vi "Config.vi"(8 "error in (no error)":errorcluster, 11 "SimSyA in":refnum<class "SimSyA.lvclass">) -> (0 "error out":errorcluster, 2 "HAL Config Data":T1, 3 "SimSyA out":refnum<class "SimSyA.lvclass">)   [LabVIEW 2014, in "SimSyA.lvlib" / "SimSyA.lvclass"]
uses:
  SimSyA.lvclass
  DriverMasterSync/build/DriverMasterSync.lvlibp/Modules/HAL/TypeDefs/HAL Config Data.ctl
  SimSyA.lvclass/SimSyA.ctl
  DriverMasterSync/build/DriverMasterSync.lvlibp/Modules/HAL/DriverMasterSync/DriverMasterSyncClass/DriverMasterSync.lvclass
  DriverMasterSync/build/DriverMasterSync.lvlibp
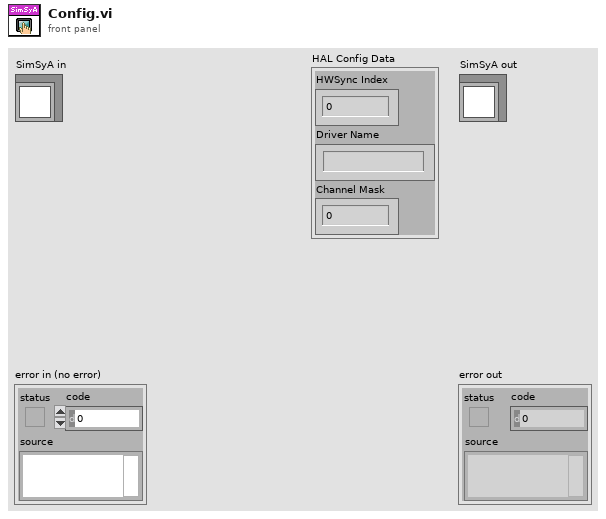
[diagram p1: front panel]
types:
  T1 = typedef "DriverMasterSync.lvlibp/HAL Config Data.ctl" = cluster{"HWSync Index":u32, "Driver Name":string, "Channel Mask":u64}
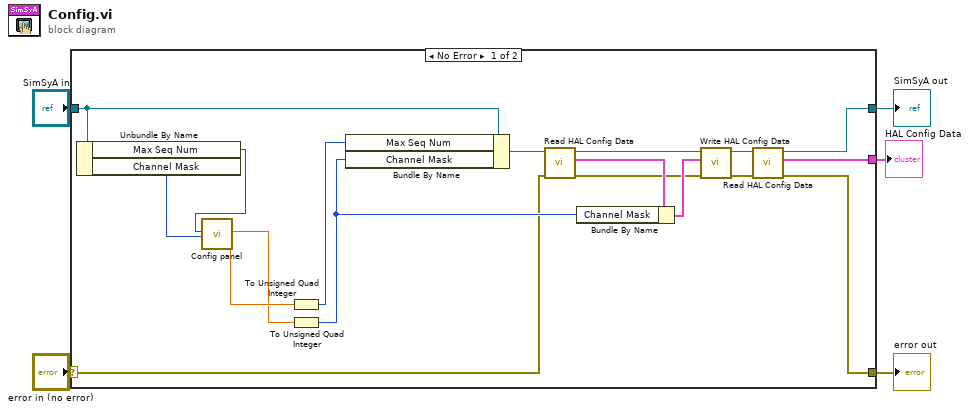
[diagram p0: block diagram]
diagram:
  n1 = case shown="No Error" "error in (no error)" {
    selector: "error in (no error)" -> [w15 w25]
    tunnel: [w10 w25] -> w4
    tunnel: [w11 w24] -> w2
    tunnel: "SimSyA in" -> [w8 w24]
    tunnel: [w9 _] -> w1
    frame No Error {
      n2 = Unbundle By Name(w8) -> ("Max Seq Num"=w7:u64, "Channel Mask"=w6:u64)
      n3 = call "Config panel.vi"("Numer of Sequences to Transfer"=w7, "Channel Mask"=w6) -> ("Channel Mask"=w22:dbl, "Numer of Sequences to Transfer"=w23:dbl)  [unwired: 14 in, 2 out]
      n4 = To Unsigned Quad Integer(1:w23) -> (0:w21:u64)
      n5 = To Unsigned Quad Integer(1:w22) -> (0:w16:u64)
      n6 = Bundle By Name(cluster=w8, "Max Seq Num"=w21, "Channel Mask"=w16) -> (w20:refnum<class "SimSyA.lvclass">)
      n7 = call "Read HAL Config Data.vi"("error in (no error)"=w15, "DriverMasterSync in"=w20) -> ("error out"=w14:errorcluster, "HAL Config Data"=w18:T1, "DriverMasterSync out"=w19:refnum<class "SimSyA.lvclass">)  [unwired: 7 in]
      n8 = Bundle By Name(cluster=w18, "Channel Mask"=w16) -> (w17:T1)
      n9 = call "Write HAL Config Data.vi"("error in (no error)"=w14, "HAL Config Data"=w17, "DriverMasterSync in"=w19) -> ("error out"=w12:errorcluster, "DriverMasterSync out"=w13:refnum<class "SimSyA.lvclass">)  [unwired: 7 in]
      n10 = call "Read HAL Config Data.vi"("error in (no error)"=w12, "DriverMasterSync in"=w13) -> ("error out"=w10:errorcluster, "HAL Config Data"=w9:T1, "DriverMasterSync out"=w11:refnum<class "SimSyA.lvclass">)  [unwired: 7 in]
    }
    frame Error {
    }
  }
  "error out" <- w4
  "SimSyA out" <- w2
  "HAL Config Data" <- w1
